vi "Close SubPanels from Map.vi"(8 "error in (no error)":errorcluster, 11 "CIF_UI in":refnum<class "CIF_UI.lvclass">) -> (0 "error out":errorcluster, 3 "CIF_UI out":refnum<class "CIF_UI.lvclass">)   [LabVIEW 2021, in "CIF_UI.lvclass"]
uses:
  CIF_UI.lvclass
  Typedef/Subpanel Map.ctl
  Typedef/Subpanel Type.ctl
  Typedef/Subpanel Data.ctl
  CIF_UI.lvclass/CIF_UI.ctl
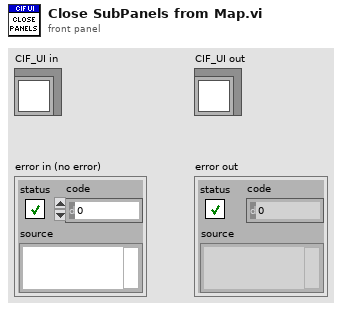
[diagram p1: front panel]
types:
  T1 = typedef "CIF_UI.lvclass/Subpanel Map.ctl" = map{T2, T3}
  T2 = typedef "CIF_UI.lvclass/Subpanel Type.ctl" = enum16{"System", "Errors", "Channel", "Plugin"}
  T3 = typedef "CIF_UI.lvclass/Subpanel Data.ctl" = cluster{"VI Reference":refnum<vi>}
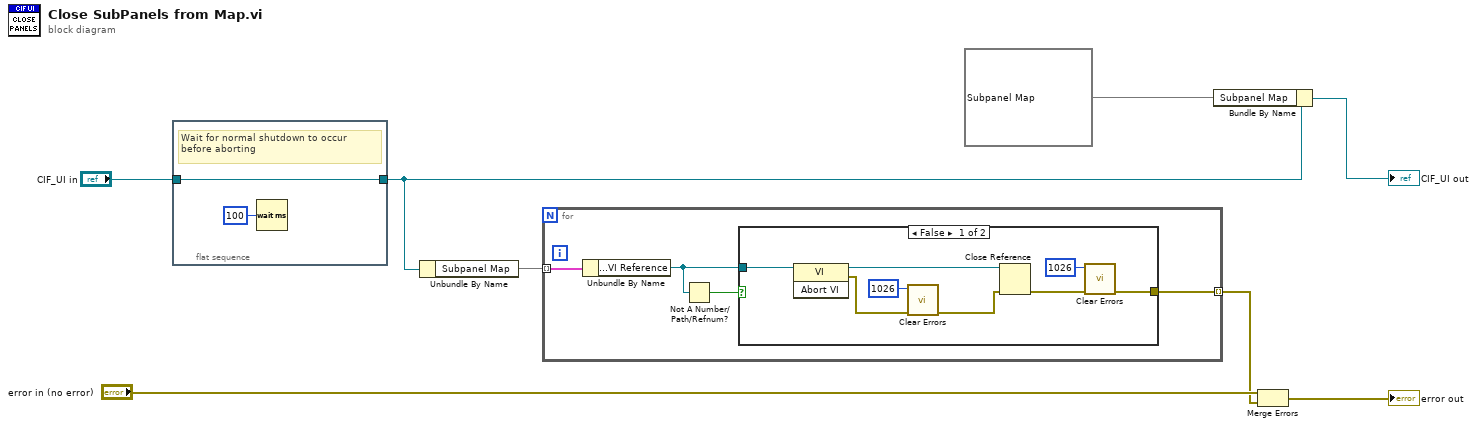
[diagram p0: block diagram]
diagram:
  n1 = flat-sequence {
    tunnel: "CIF_UI in" -> [w9]
    tunnel: [w9] -> w1
    frame #0 {
      # "Wait for normal shutdown to occur before aborting"
      n2 = Wait (ms)(milliseconds to wait=u32 100) -> ()  [unwired: 1 out]
    }
  }
  n3 = Unbundle By Name(w1) -> ("Subpanel Map"=w6:T1)
  n4 = for {
    tunnel: w6 -> [w14] mode=indexing
    tunnel: [w11] -> w4 mode=indexing
    n5 = Unbundle By Name(w14) -> ("SubPanel Data.VI Reference"=w12:refnum<vi>)
    n6 = Not A Number/Path/Refnum?(number/path/refnum=w12) -> (NaN/Path/Refnum?=w13:bool)
    n7 = case shown="False" w13 {
      tunnel: w12 -> [w22 _]
      tunnel: [w15 _] -> w11
      frame False {
        n8 = invoke class="VI" method="Abort VI"(reference=w22) -> (reference out=w21:refnum<vi>, error out=w19:errorcluster)  [unwired: 2 in, 1 out]
        n9 = call <vilib>:"Clear Errors.vi"("error in (no error)"=w19, "specific error code to clear (0: all)"=1026) -> ("error out"=w18:errorcluster)  [unwired: 4 in, 1 out]
        n10 = Close Reference(reference=w21, error in (no error)=w18) -> (error out=w16:errorcluster)
        n11 = call <vilib>:"Clear Errors.vi"("error in (no error)"=w16, "specific error code to clear (0: all)"=1026) -> ("error out"=w15:errorcluster)  [unwired: 4 in, 1 out]
      }
      frame True {
      }
    }
  }
  n12 = Bundle By Name(cluster=w1, "Subpanel Map"=T1 {}) -> (→"CIF_UI out":refnum<class "CIF_UI.lvclass">)
  n13 = Merge Errors("error in (no error)", w4) -> (→"error out":errorcluster)
